vi "Acquire Data.vi"() -> ()   [LabVIEW 2011]
uses:
  <vilib>/Motion/FlexMotion/FunctionsVIs/Trajectory.llb/Acquire Trajectory Data (8 axes).flx
panel:
  out "Axis 2 Velocity":i32[](array[numeric])
  out "Axis 2 Position":i32[](array[numeric])
  out "Axis 1 Velocity":i32[](array[numeric])
  out "Axis 1 Position":i32[](array[numeric])
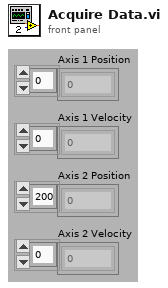
[diagram p1: front panel]
types:
  T1 = cluster{bool, bool, bool, bool, bool, bool, bool, bool}
  T2 = typedef "Board Id" = u8
  T3 = typedef "Bd Id Out" = u8
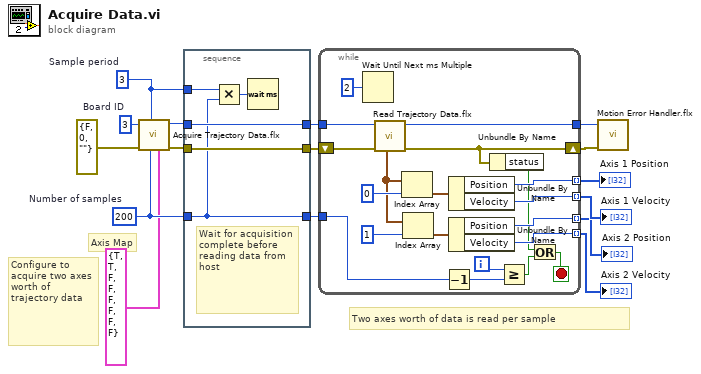
[diagram p0: block diagram]
diagram:
  w6 = u16 200  # Number of samples
  w7 = u16 3  # Sample period
  w2 = T2 3  # Board ID
  # "Axis Map"
  # "Configure to acquire two axes worth of trajectory data"
  # "Two axes worth of data is read per sample"
  n1 = call-poly <vilib>:"Acquire Trajectory Data.flx"("Axis Map (Disabled)"=T1 {TRUE, TRUE, FALSE, FALSE, FALSE, FALSE, FALSE, FALSE}, "Number of samples (1)"=w6, "Timeperiod (3 ms)"=w7, "error in (no error)"=errorcluster {"status"=FALSE, "code"=0, "source"=""}, "Board ID"=w2) -> ("error out"=w3:errorcluster, "Bd ID Out"=w4:T3)  [unwired: 5 in]
  n2 = stacked-sequence {
    tunnel: [w21] -> w10
    tunnel: w3 -> [w21]
    tunnel: [w20] -> w9
    tunnel: w4 -> [w20]
    tunnel: w7 -> [w19]
    tunnel: w6 -> [w17]
    tunnel: [w17] -> w8
    frame #0 {
      # "Wait for acquisition complete before reading data from host"
      n3 = Multiply(x=w19, y=w17) -> (x*y=w18:u16)
      n4 = Wait (ms)(milliseconds to wait=w18) -> ()  [unwired: 1 out]
    }
  }
  n5 = while {
    tunnel: w8 -> [w22]
    tunnel: [w30] -> w11 mode=indexing
    tunnel: [w31] -> w12 mode=indexing
    tunnel: [w32] -> w13 mode=indexing
    tunnel: [w33] -> w14 mode=indexing
    tunnel: [w39] -> w15
    shift-left: w10 -> [w40]
    shift-right: [w26] -> w16
    tunnel: w9 -> [w41]
    i -> [w29]
    stop <- w27 stop-if-true
    n6 = Wait Until Next ms Multiple(millisecond multiple=u32 2) -> ()  [unwired: 1 out]
    n7 = call <vilib>:"Read Trajectory Data.flx"("error in (no error)"=w40, "Board ID"=w41) -> ("error out"=w26:errorcluster, "Bd ID Out"=w39:T3, "Sample Data"=w36:cluster{"Position":i32, "Velocity":i32}[])  [unwired: 4 in]
    n8 = Index Array(array=w36, index=0) -> (element=w35:cluster{"Position":i32, "Velocity":i32})
    n9 = Index Array(array=w36, index=1) -> (element=w34:cluster{"Position":i32, "Velocity":i32})
    n10 = Decrement(x=w22) -> (x-1=w23:u16)
    n11 = Unbundle By Name(w35) -> ("Position"=w33:i32, "Velocity"=w32:i32)
    n12 = Unbundle By Name(w34) -> ("Position"=w31:i32, "Velocity"=w30:i32)
    n13 = Unbundle By Name(w26) -> ("status"=w25:bool)
    n14 = Greater Or Equal?(x=w29, y=w23) -> (x >= y?=w28:bool)
    n15 = Or(x=w25, y=w28) -> (x .or. y?=w27:bool)
  }
  "Axis 1 Position" <- w14
  "Axis 1 Velocity" <- w13
  "Axis 2 Position" <- w12
  "Axis 2 Velocity" <- w11
  n16 = call <vilib>:"Motion Error Handler.flx"("Board ID"=w15, "error in (no error)"=w16) -> ()  [unwired: 9 in, 5 out]
